vi "Read FC1 Force Sensor.vi"(8 "error in (no error)":errorcluster, 11 "Model in":refnum<class "Model.lvclass">) -> (0 "error out":errorcluster, 3 "Model out":refnum<class "Model.lvclass">)   [LabVIEW 2015, in "Model.lvclass"]
uses:
  Model.lvclass
  ILC ADC/ILC ADC Factory/ILC ADC Factory.lvclass
  Model.lvclass/Model.ctl
  ILC ADC/ILC ADC/ILC ADC.lvclass
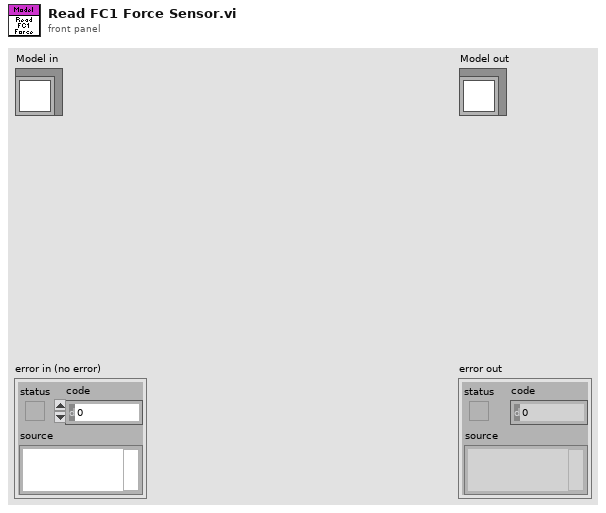
[diagram p1: front panel]
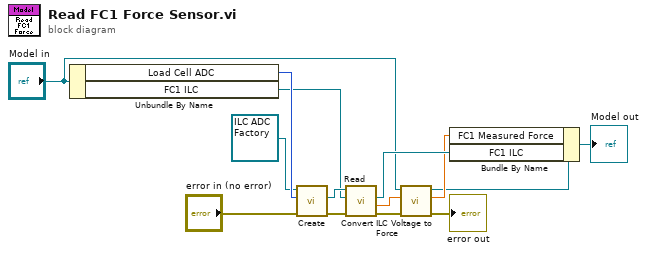
[diagram p0: block diagram]
diagram:
  n1 = Unbundle By Name("Model in") -> ("Load Cell ADC"=w14:u8, "FC1 ILC"=w12:refnum<class "ILC.lvclass">)
  n2 = call-dynamic "Create.vi"("error in (no error)"="error in (no error)", "Channel"=w14, "ILC ADC Factory in"=refnum<class "ILC ADC Factory.lvclass"> refnum ("ILCADCFactory in")) -> ("error out"=w7:errorcluster, "ILC ADC"=w13:refnum<class "ILC ADC.lvclass">)  [unwired: 6 in, 1 out]
  n3 = call-dynamic "Read.vi"("error in (no error)"=w7, "ILC In"=w12, "ILC ADC in"=w13) -> ("error out"=w6:errorcluster, "Value"=w8:dbl[unit], "ILC Out"=w11:refnum<class "ILC.lvclass">)  [unwired: 5 in, 1 out]
  n4 = call "Convert ILC Voltage to Force.vi"("error in (no error)"=w6, "Voltage"=w8, "Model in"="Model in") -> ("error out"=→"error out":errorcluster, "Force"=w4:dbl[unit], "Model out"=w2:refnum<class "Model.lvclass">)  [unwired: 6 in]
  n5 = Bundle By Name(cluster=w2, "FC1 Measured Force"=w4, "FC1 ILC"=w11) -> (→"Model out":refnum<class "Model.lvclass">)
